vi "Door_current.vi"(0 "Strings in":string[](array[string])=["C:\\CuspControl\\GPIB and Network\\Cusp\\Dummyfile.txt", "6723"], 1 "Dubs in":dbl[](array[numeric])=[0.0]) -> ()   [LabVIEW 2018]
uses:
  <vilib>/Analysis/1siggen.llb/Ramp Pattern by Samples.vi
  <vilib>/DAQmx/write.llb/DAQmx Write (Analog DBL 1Chan 1Samp).vi
  <vilib>/DAQmx/create/channels.llb/DAQmx Create Channel (AO-Voltage-Basic).vi
  <vilib>/DAQmx/miscellaneous.llb/DAQmx Fill In Error Info.vi
  <vilib>/Analysis/NI_AALBase.lvlib
panel:
  out "Elapsed time (ms)":u32=37
  out "Ramp Pattern":dbl[](array[numeric])=[1.0, 0.9583333333333334, 0.9166666666666666, 0.875, 0.8333333333333334, 0.7916666666666667, 0.75, 0.7083333333333334, 0.6666666666666667, 0.625, 0.5833333333333334, 0.5416666666666667, 0.5, 0.45833333333333337, 0.41666666666666674, 0.375, 0.33333333333333337, 0.29166666666666674, 0.25, 0.20833333333333337, 0.16666666666666674, 0.125, 0.08333333333333337, 0.04166666666666674, 0.0]
  in  "samples":i32=25
  in  "file (use dialog)":path=path "C:/CuspControl/GPIB and Network/Cusp/DoorVolts.txt"
  in  "subvi":bool=TRUE
  out "error out":errorcluster
  in  "AO2 name":string="6723"
  in  "Takasago Vc ao line":string="/ao12"
  in  "ON voltage":dbl format="%#_13g"
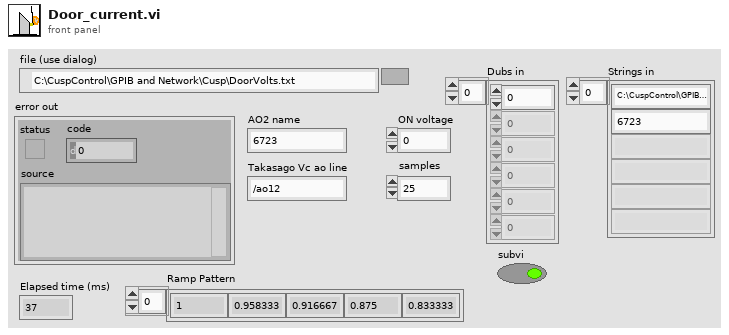
[diagram p1: front panel]
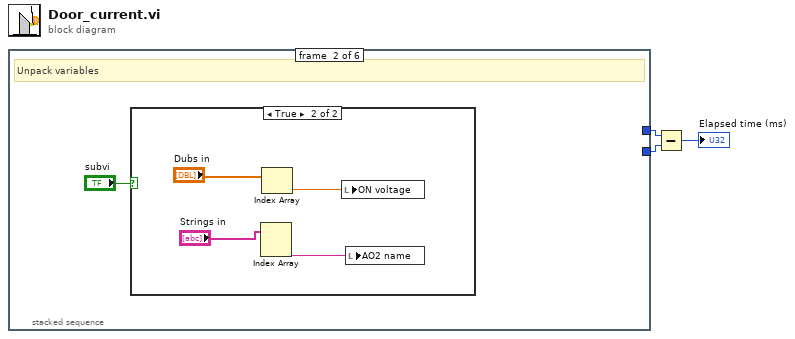
[diagram p0: block diagram]
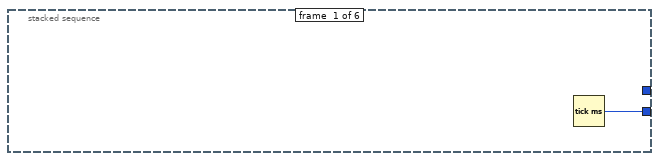
[diagram p2: hidden frame]
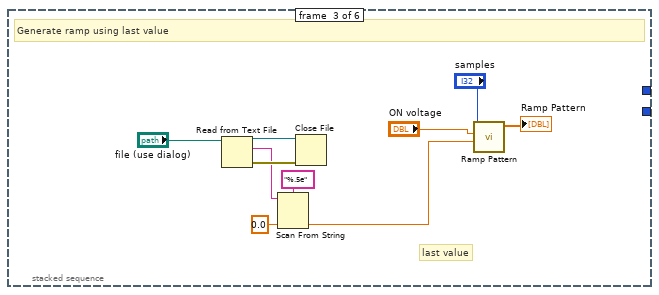
[diagram p4: hidden frame]
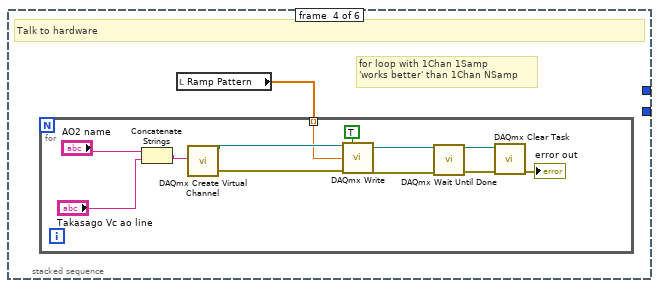
[diagram p5: hidden frame]
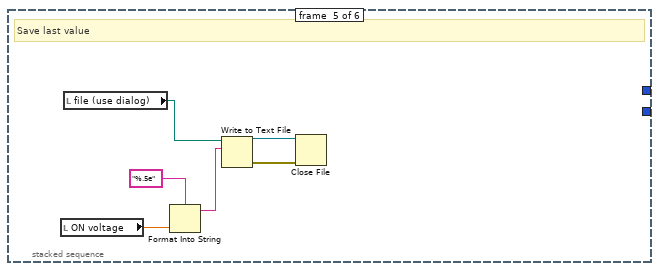
[diagram p6: hidden frame]
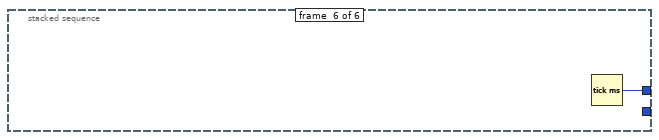
[diagram p7: hidden frame]
diagram:
  n1 = stacked-sequence {
    tunnel: [w4 _ _ _ _ _] -> w2
    tunnel: [_ _ _ _ _ w39] -> w3
    frame #0 {
      n2 = Tick Count (ms)() -> (millisecond timer value=w4:u32)
    }
    frame #1 {
      # "Unpack variables"
      n3 = case shown="True" "subvi" {
        frame False {
        }
        frame True {
          n4 = Index Array(array="Strings in") -> (element #2=w6:string)  [unwired: 2 in, 1 out]
          n5 = Index Array(array="Dubs in") -> (element=w7:dbl)  [unwired: 1 in]
          n6 = local write "ON voltage"(w7) -> ()
          n7 = local write "AO2 name"(w6) -> ()
        }
      }
    }
    frame #2 {
      # "last value"
      # "Generate ramp using last value"
      n8 = Read from Text File(file (use dialog)="file (use dialog)") -> (refnum out=w18:refnum<file>, text=w16:string, error out=w17:errorcluster)  [unwired: 3 in, 1 out]
      n9 = Scan From String(format string="%.5e", input string=w16, default 1=0.0 ("default value 1")) -> (output 1=w13:dbl)  [unwired: 2 in, 3 out]
      n10 = Close File(refnum=w18, error in=w17) -> ()  [unwired: 2 out]
      n11 = call-poly <vilib>:"Ramp Pattern.vi"("start"=w13, "end"="ON voltage", "samples"="samples") -> ("Ramp Pattern"=→"Ramp Pattern":dbl[])  [unwired: 7 in, 1 out]
    }
    frame #3 {
      # "for loop with 1Chan 1Samp \n'works better' than 1Chan NSamp"
      # "Talk to hardware"
      n12 = local read "Ramp Pattern"() -> (w20:dbl[])
      n13 = for {
        tunnel: w20 -> [w22] mode=indexing
        n14 = Concatenate Strings("AO2 name", "Takasago Vc ao line") -> (w28:string)
        n15 = call-poly <vilib>:"DAQmx Create Virtual Channel.vi"("physical channels"=w28) -> ("task out"=w24:refnum<k21>, "error out"=w23:errorcluster)  [unwired: 13 in]
        n16 = call-poly <vilib>:"DAQmx Write.vi"("task/channels in"=w24, "auto start"=TRUE, "data"=w22, "error in"=w23) -> ("task out"=w30:refnum<k21>, "error out"=w29:errorcluster)  [unwired: 9 in, 1 out]
        n17 = call <vilib>:"DAQmx Wait Until Done.vi"("task/channels in"=w30, "error in"=w29) -> ("task out"=w32:refnum<k21>, "error out"=w31:errorcluster)  [unwired: 12 in]
        n18 = call <vilib>:"DAQmx Clear Task.vi"("task in"=w32, "error in"=w31) -> ("error out"=→"error out":errorcluster)  [unwired: 13 in]
      }
    }
    frame #4 {
      # "Save last value"
      n19 = local read "ON voltage"() -> (w35:dbl)
      n20 = local read "file (use dialog)"() -> (w36:path)
      n21 = Format Into String(format string="%.5e", w35) -> (resulting string=w34:string)  [unwired: 2 in, 1 out]
      n22 = Write to Text File(file (use dialog)=w36, text=w34) -> (refnum out=w38:refnum<file>, error out=w37:errorcluster)  [unwired: 2 in, 1 out]
      n23 = Close File(refnum=w38, error in=w37) -> ()  [unwired: 2 out]
    }
    frame #5 {
      n24 = Tick Count (ms)() -> (millisecond timer value=w39:u32)
    }
  }
  n25 = Subtract(x=w3, y=w2) -> (x-y=→"Elapsed time (ms)":u32)
